vi "main screen queue out Unitest.vi"(8 "error in (no error)":errorcluster) -> (0 "error out":errorcluster, 3 "output Queue":T1)   [LabVIEW 2025]
uses:
  C:/LAB-IQ/B2V2/WO 2470/support/init queue out loop.ctl
  LAB-IQ/B2V2/WO 2470/v01/support/Message Queue/Message Cluster.ctl
  REF Enum Unitest.ctl
  LAB-IQ/B2V2/WO 2470/v01/support/Message Queue/Message Queue.lvlib
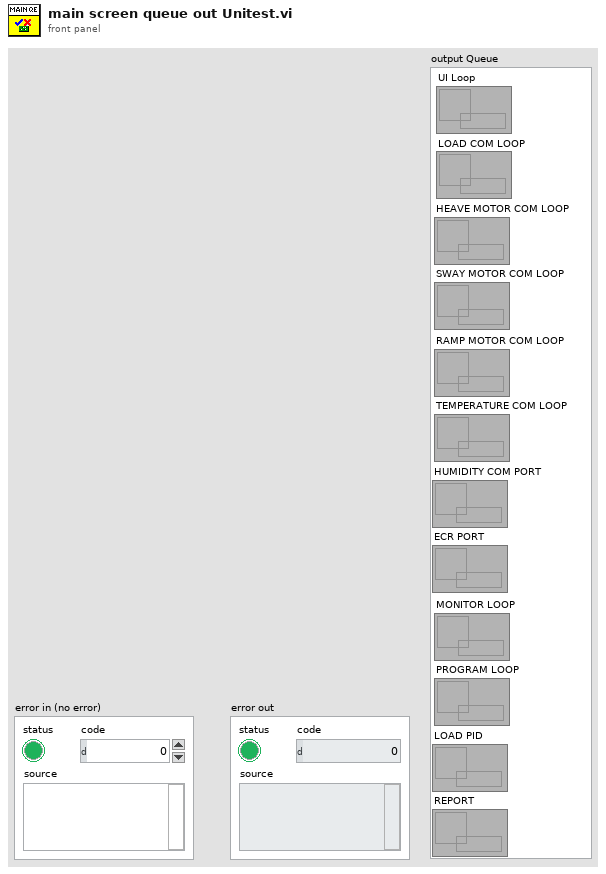
[diagram p1: front panel]
types:
  T1 = typedef "init queue out loop.ctl" = cluster{"UI Loop":refnum<queue>, "LOAD COM LOOP ":refnum<queue>, "SWAY MOTOR COM LOOP":refnum<queue>, "HEAVE MOTOR COM LOOP":refnum<queue>, "TEMPERATURE COM LOOP":refnum<queue>, "RAMP MOTOR COM LOOP":refnum<queue>, "ECR PORT":refnum<queue>, "HUMIDITY COM PORT":refnum<queue>, "PROGRAM LOOP":refnum<queue>, "MONITOR LOOP":refnum<queue>, "REPORT":refnum<queue>, "LOAD PID":refnum<queue>}
  T2 = typedef "REF Enum Unitest.ctl" = enum16{"Init", "UI Loop", "LOAD COM LOOP", "HEAVE MOTOR COM LOOP", "SWAY MOTOR COM LOOP", "RAMP MOTOR COM LOOP", "TEMPERATURE COM LOOP", "HUMIDITY COM PORT", "ECR PORT", "MONITOR LOOP", "PROGRAM LOOP", "LOAD PID", "REPORT"}
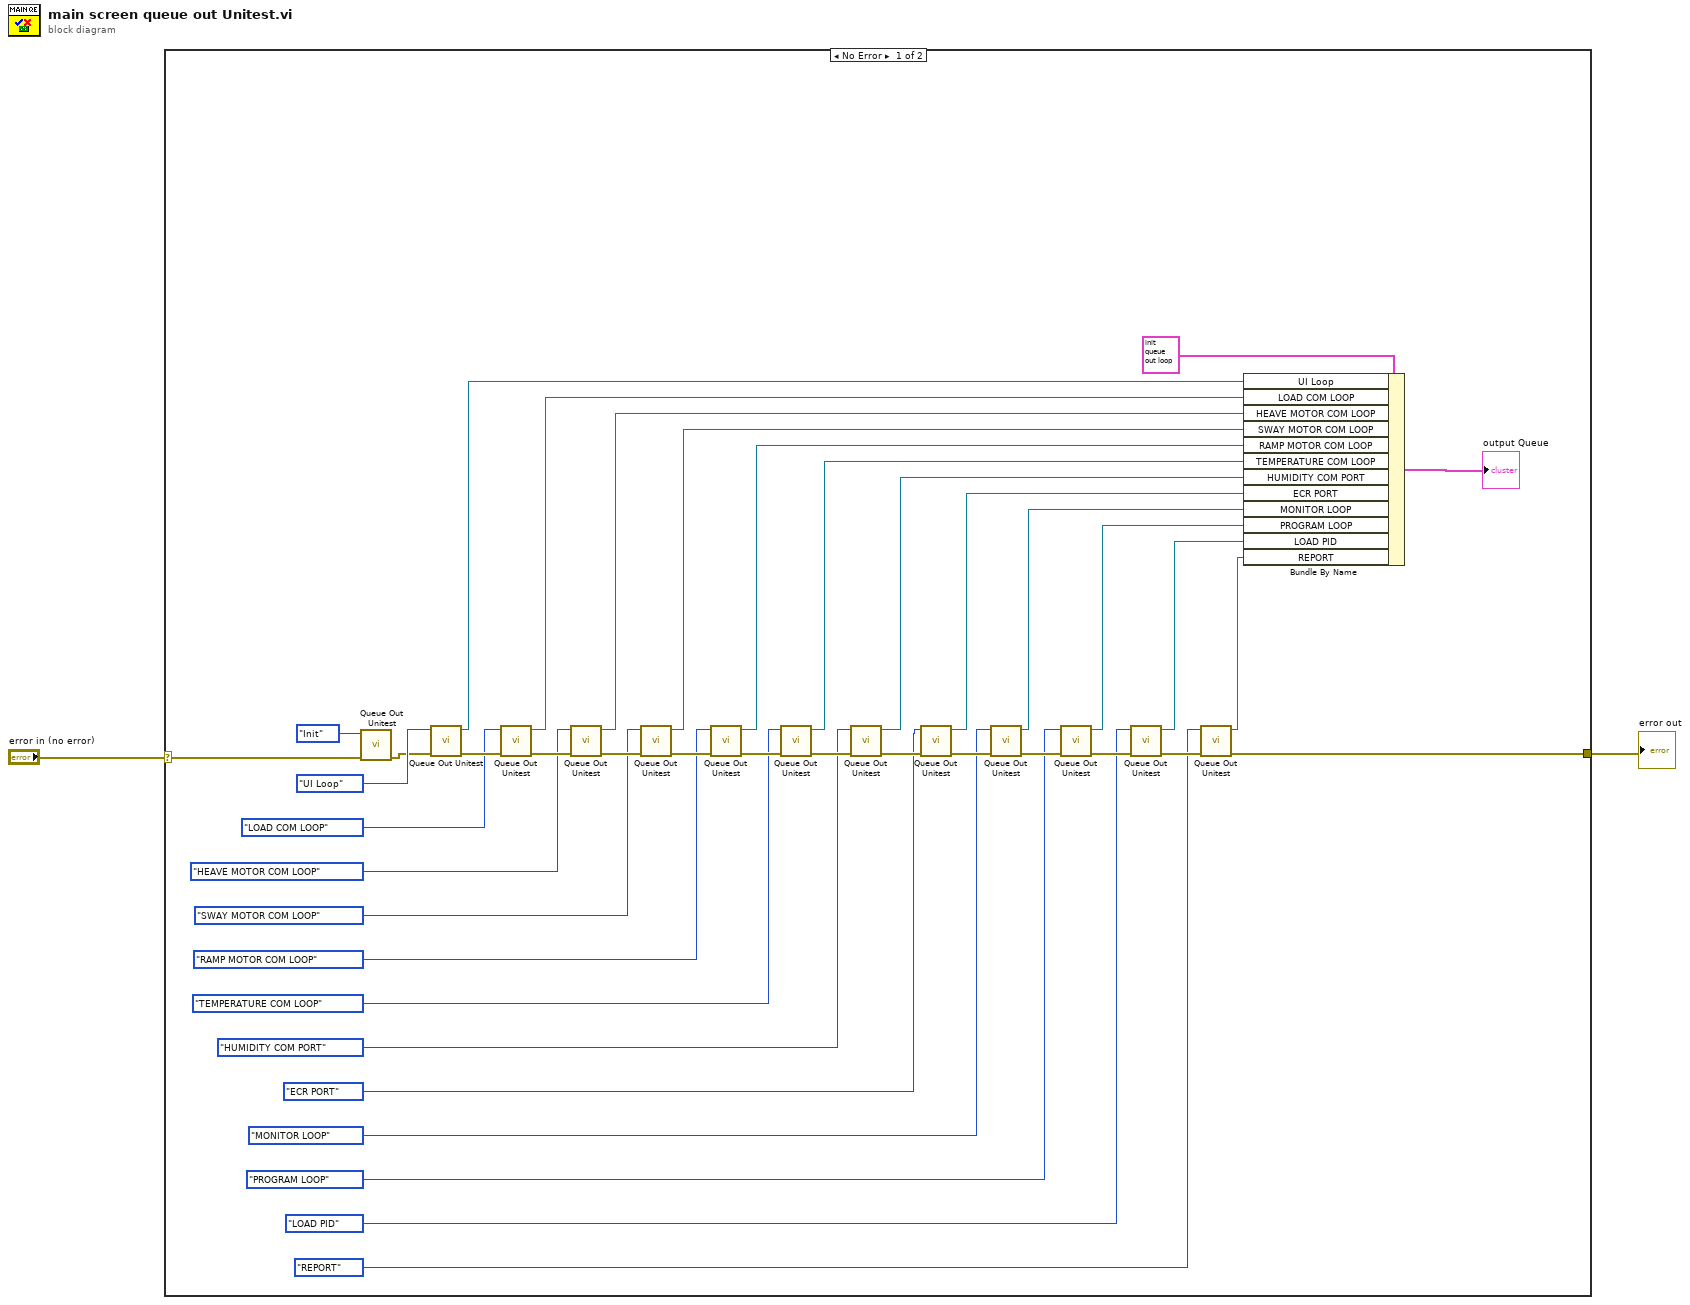
[diagram p0: block diagram]
diagram:
  n1 = case shown="No Error" "error in (no error)" {
    selector: "error in (no error)" -> [w41 _]
    tunnel: [w26 _] -> w2
    frame No Error {
      n2 = call "Queue Out Unitest.vi"("error in"=w41, 11:REF_Enum_Unitest."Init") -> ("error out"=w38:errorcluster)  [unwired: 8 in, 1 out]
      n3 = call "Queue Out Unitest.vi"("error in"=w38, 11:REF_Enum_Unitest."UI Loop") -> ("error out"=w37:errorcluster, "Queue Out"=w25:refnum<queue>)  [unwired: 8 in]
      n4 = call "Queue Out Unitest.vi"("error in"=w37, 11:REF_Enum_Unitest."LOAD COM LOOP") -> ("error out"=w36:errorcluster, "Queue Out"=w24:refnum<queue>)  [unwired: 8 in]
      n5 = call "Queue Out Unitest.vi"("error in"=w36, 11:REF_Enum_Unitest."HEAVE MOTOR COM LOOP") -> ("error out"=w35:errorcluster, "Queue Out"=w23:refnum<queue>)  [unwired: 8 in]
      n6 = call "Queue Out Unitest.vi"("error in"=w35, 11:REF_Enum_Unitest."SWAY MOTOR COM LOOP") -> ("error out"=w34:errorcluster, "Queue Out"=w22:refnum<queue>)  [unwired: 8 in]
      n7 = call "Queue Out Unitest.vi"("error in"=w34, 11:REF_Enum_Unitest."RAMP MOTOR COM LOOP") -> ("error out"=w33:errorcluster, "Queue Out"=w21:refnum<queue>)  [unwired: 8 in]
      n8 = call "Queue Out Unitest.vi"("error in"=w33, 11:REF_Enum_Unitest."TEMPERATURE COM LOOP") -> ("error out"=w32:errorcluster, "Queue Out"=w20:refnum<queue>)  [unwired: 8 in]
      n9 = call "Queue Out Unitest.vi"("error in"=w32, 11:REF_Enum_Unitest."HUMIDITY COM PORT") -> ("error out"=w31:errorcluster, "Queue Out"=w19:refnum<queue>)  [unwired: 8 in]
      n10 = call "Queue Out Unitest.vi"("error in"=w31, 11:REF_Enum_Unitest."ECR PORT") -> ("error out"=w30:errorcluster, "Queue Out"=w18:refnum<queue>)  [unwired: 8 in]
      n11 = call "Queue Out Unitest.vi"("error in"=w30, 11:REF_Enum_Unitest."MONITOR LOOP") -> ("error out"=w29:errorcluster, "Queue Out"=w17:refnum<queue>)  [unwired: 8 in]
      n12 = call "Queue Out Unitest.vi"("error in"=w29, 11:REF_Enum_Unitest."PROGRAM LOOP") -> ("error out"=w28:errorcluster, "Queue Out"=w16:refnum<queue>)  [unwired: 8 in]
      n13 = call "Queue Out Unitest.vi"("error in"=w28, 11:REF_Enum_Unitest."LOAD PID") -> ("error out"=w27:errorcluster, "Queue Out"=w15:refnum<queue>)  [unwired: 8 in]
      n14 = call "Queue Out Unitest.vi"("error in"=w27, 11:REF_Enum_Unitest."REPORT") -> ("error out"=w26:errorcluster, "Queue Out"=w14:refnum<queue>)  [unwired: 8 in]
      n15 = Bundle By Name(cluster=T1 {"UI Loop"=refnum, "LOAD COM LOOP "=refnum, "SWAY MOTOR COM LOOP"=refnum, "HEAVE MOTOR COM LOOP"=refnum, "TEMPERATURE COM LOOP"=refnum, "RAMP MOTOR COM LOOP"=refnum, "ECR PORT"=refnum, "HUMIDITY COM PORT"=refnum, "PROGRAM LOOP"=refnum, "MONITOR LOOP"=refnum, "REPORT"=refnum, "LOAD PID"=refnum}, "UI Loop"=w25, "LOAD COM LOOP"=w24, "HEAVE MOTOR COM LOOP"=w23, "SWAY MOTOR COM LOOP"=w22, "RAMP MOTOR COM LOOP"=w21, "TEMPERATURE COM LOOP"=w20, "HUMIDITY COM PORT"=w19, "ECR PORT"=w18, "MONITOR LOOP"=w17, "PROGRAM LOOP"=w16, "LOAD PID"=w15, "REPORT"=w14) -> (→"output Queue":T1)
    }
    frame Error {
    }
  }
  "error out" <- w2
